vi "PI Convert 1.4 to 1.5.vi"(0 "Prompted Inputs 1.4 Test Parameters":T3) -> (1 "Datasheets":T1, 2 "Prompted Inputs 1.5 Test Parameters":T2)   [LabVIEW 2011]
uses:
  TypeDefs/PI Test Parameters v1.4.ctl
  TypeDefs/PI Test Parameters v1.5.ctl
  Test Datasheets v1.0-4.0.ctl
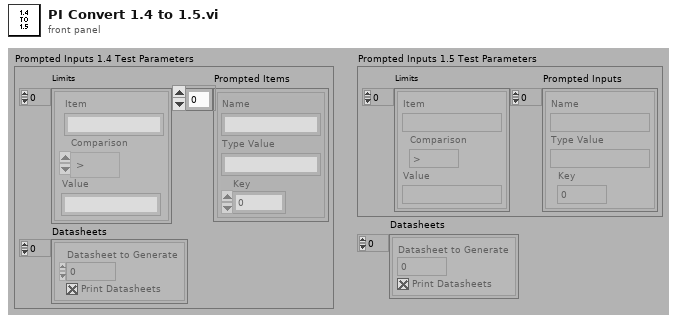
[diagram p1: front panel]
types:
  T1 = typedef "Test Datasheets v1.0-4.0.ctl" = cluster{"Datasheet to Generate":i32, "Print Datasheets":bool}[]
  T2 = typedef "PI Test Parameters v1.5.ctl" = cluster{"Limits":cluster{"Item":string, "Comparison":enum16{">", ">=", "<", "<=", "<>", "="}, "Value":string}[], "Prompted Inputs":cluster{"Name":string, "Type Value":string, "Key":i32}[]}
  T3 = typedef "PI Test Parameters v1.4.ctl" = cluster{"Limits":cluster{"Item":string, "Comparison":enum16{">", ">=", "<", "<=", "<>", "="}, "Value":string}[], "Datasheets":cluster{"Datasheet to Generate":i32, "Print Datasheets":bool}[], "Prompted Items":cluster{"Name":string, "Type Value":string, "Key":i32}[]}
  T4 = cluster{"Item":string, "Comparison":enum16{">", ">=", "<", "<=", "<>", "="}, "Value":string}[]
  T5 = cluster{"Name":string, "Type Value":string, "Key":i32}[]
  T6 = cluster{"Datasheet to Generate":i32, "Print Datasheets":bool}[]
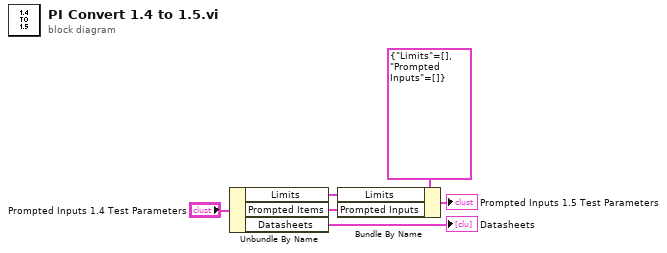
[diagram p0: block diagram]
diagram:
  n1 = Unbundle By Name("Prompted Inputs 1.4 Test Parameters") -> ("Limits"=w5:T4, "Prompted Items"=w2:T5, "Datasheets"=→"Datasheets":T6)
  n2 = Bundle By Name(cluster=T2 {"Limits"=[], "Prompted Inputs"=[]} ("Prompted Inputs Test Parameters"), "Limits"=w5, "Prompted Inputs"=w2) -> (→"Prompted Inputs 1.5 Test Parameters":T2)
